vi "Get 1D String.vi"(5 "format string (%s)":string="%s", 7 "key description":string, 8 "sections":string[](array[string]), 9 "string":string[](array[string]), 11 "info data":string) -> (0 "sections out":string[](array[string]), 2 "value":string[](array[string]), 3 "info data out":string)   [LabVIEW 2019, in "infolib.lvlib"]
doc: "Reads horizontal or vertical vector of strings. If section is entered it searches the key in the section(s)."
uses:
  infolib.lvlib
  Get 2D String.vi
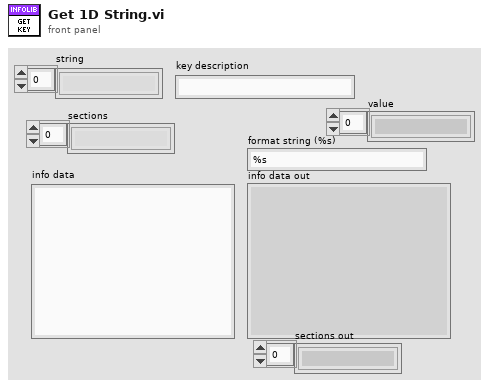
[diagram p1: front panel]
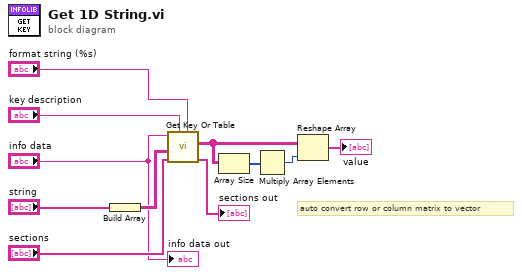
[diagram p0: block diagram]
diagram:
  # "auto convert row or column matrix to vector"
  n1 = Build Array("string") -> (w7:string[][])
  n2 = call-poly "Get Key Or Table.vi"("format string (%s)"="format string (%s)", "key description"="key description", "sections"="sections", "string"=w7, "info data"="info data") -> ("sections out"=→"sections out":string[], "value"=w2:string[][])  [unwired: 4 in, 1 out]
  n3 = Array Size(array=w2) -> (size(s)=w11:i32[])
  n4 = Multiply Array Elements(1:w11) -> (0:w10:i32)
  n5 = Reshape Array(w2, w10) -> (→"value":string[])
  "info data out" <- "info data"
